vi "test BC + RTs.vi"(8 "error in":errorcluster, 11 "TestCase in":refnum<class "Create Execution Unit.lvclass">) -> (0 "error out":errorcluster, 3 "TestCase out":refnum<class "Create Execution Unit.lvclass">)   [LabVIEW 2023, in "Create Execution Unit.lvclass"]
uses:
  Create Execution Unit.lvclass
  C:/Program Files/National Instruments/LabVIEW 2023/vi.lib/NI/VeriStand Custom Device Testing Tools/VeriStandScriptingTestCase/VeriStandScriptingTestCase.lvclass
  Shared/Map of Messages to Value Indexes.ctl
  Shared/Message Map Key.ctl
  Engine/Implementation/Rx Execution Unit/Message Map Value.ctl
  Shared/Message Definition.ctl
  Shared/Message Type.ctl
  Shared/Terminal Endpoint.ctl
  Shared/Address.ctl
  Shared/Parameter Definition.ctl
  Engine/Implementation/Execution Unit Factory/Execution Unit Factory.lvclass
  Engine/Implementation/Rx Execution Unit/Rx Execution Unit.lvclass
  Engine/Custom Device/Logging Configuration.ctl
  Shared/Data Word Format.ctl
  Shared/Device Parameters.ctl
  Shared/Initialization Method.ctl
  <vilib>/NI/VeriStand Custom Device Testing Tools/VeriStandScriptingTestCase/VeriStandScriptingTestCase.lvclass/VeriStandScriptingTestCase.ctl
  Engine/Implementation/Rx Execution Unit/Rx Execution Unit.lvclass/Rx Execution Unit.ctl
  <vilib>/NI/VeriStand Custom Device Testing Tools/VeriStandScriptingTestCase/Read Target.vi
  Engine/Implementation/Shared Resources/Shared Resources.lvclass
  C:/dev/niveristand-ballard-milStd1553-custom-device/Source/Custom Device Support/Engine/Interfaces/Shared Resources/Shared Resources.lvclass
  NationalInstruments.VeriStand.SystemDefinitionAPI
  Create Execution Unit.lvclass/Create Execution Unit.ctl
  <vilib>/addons/_JKI Toolkits/VI Tester/TestCase.llb/TestCase.lvclass
  Scripting/Ballard MIL-STD-1553 Scripting.lvlib
  Engine/Custom Device/Custom Device.lvlib
  C:/Program Files/National Instruments/LabVIEW 2023/vi.lib/addons/_JKI Toolkits/VI Tester/TestCase.llb/TestCase.lvclass
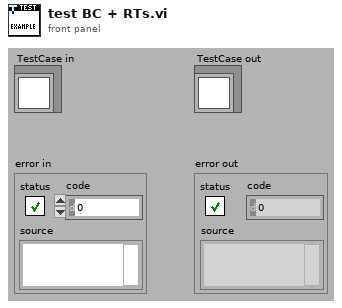
[diagram p1: front panel]
types:
  T1 = typedef "Map of Messages to Value Indexes.ctl" = map{T2, T3}
  T2 = typedef "Message Map Key.ctl" = cluster{"HW channel":u16, "terminal address":u16, "subaddress":u16, "mode code":u16}
  T3 = typedef "Ballard MIL-STD-1553 Engine Support.lvlib/Implementation.lvlib/Rx Execution Unit.lvclass/Message Map Value.ctl" = cluster{"value indexes":i32[], "message":T4, "Tx status count":i32, "Rx status count":i32}
  T4 = typedef "Message Definition.ctl" = cluster{"name":string, "message type":T5, "endpoint Tx":T6, "endpoint Rx":T6, "create timestamp channel":bool, "mode code":u16, "number of words":u16, "parameters":cluster{"name":string, "default value":dbl, "unit":string, "parameter definition":T8}[]}
  T5 = typedef "Message Type.ctl" = string
  T6 = typedef "Terminal Endpoint.ctl" = cluster{"terminal address":T7, "subaddress":T7}
  T7 = typedef "Address.ctl" = u16
  T8 = typedef "Parameter Definition.ctl" = cluster{"start index":i32, "size (bits)":i32, "encoding":enum16{"BNR", "BCD", "Discrete"}, "signed":bool, "multiplier":dbl, "offset":dbl}
  T9 = typedef "Device Parameters.ctl" = cluster{"initialization method":T10, "card number":i32, "PXI slot number":i32, "core number":i32}
  T10 = typedef "Initialization Method.ctl" = enum16{"PXI Slot Number", "Card Number"}
  T11 = typedef "Ballard MIL-STD-1553 Engine Support.lvlib/Custom Device.lvlib/Logging Configuration.ctl" = cluster{"configured":bool, "directory":string, "file name":string, "timestamp file name":bool, "data word format":T12}
  T12 = typedef "Data Word Format.ctl" = string
  T13 = cluster{"Hardware File":path, "Parameters File":path}
  T14 = typedef "Custom Device API.lvlib/Custom Device Item Ref.ctl" = u64
  T15 = typedef "Ballard MIL-STD-1553 Engine Support.lvlib/Interfaces.lvlib/Execution Unit Information.ctl" = cluster{"Execution Unit":refnum<class "Execution Unit.lvclass">, "Incoming Channels":T14[], "Outgoing Channels":T14[], "ReadWrite Channels":T14[]}
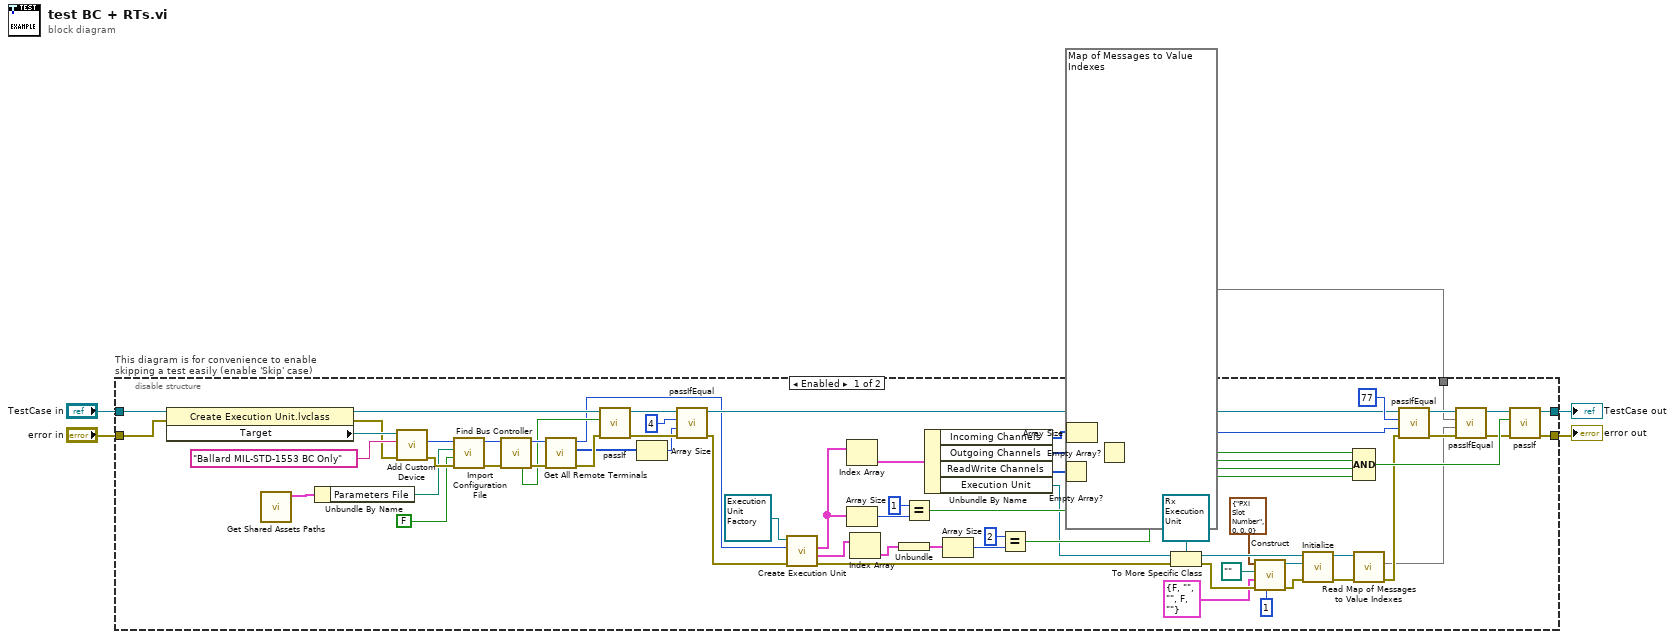
[diagram p0: block diagram]
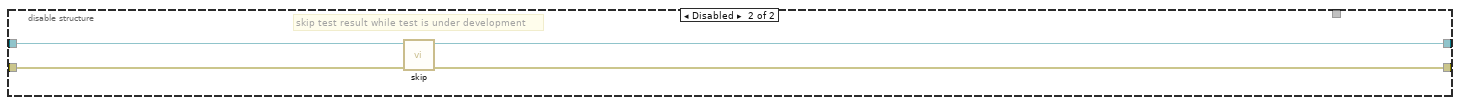
[diagram p2: hidden frame]
diagram:
  n1 = disable-structure "This diagram is for convenience to enable skipping a test easily (enable 'Skip' case)" shown="Enabled" {
    disable-tunnel: "TestCase in" -> [w67 w76]
    disable-tunnel: [w42 w74] -> w2
    disable-tunnel: [w41 w75] -> w4
    disable-tunnel: "error in" -> [w71 w73]
    disable-tunnel: T1 {{"HW channel"=0, "terminal address"=0, "subaddress"=2, "mode code"=0}={"value indexes"=[0], "message"={"name"="BC to RT 0.2", "message type"="BC to RT", "endpoint Tx"={"terminal address"=99, "subaddress"=0}, "endpoint Rx"={"terminal address"=0, "subaddress"=2}, "create timestamp channel"=TRUE, "mode code"=0, "number of words"=3, "parameters"=[{"name"="Word 00", "default value"=0.0, "unit"="", "parameter definition"={"start index"=0, "size (bits)"=16, "encoding"=enum."BNR", "signed"=FALSE, "multiplier"=1.0, "offset"=0.0}}, {"name"="Word 01", "default value"=0.0, "unit"="", "parameter definition"={"start index"=16, "size (bits)"=16, "encoding"=enum."BNR", "signed"=FALSE, "multiplier"=1.0, "offset"=0.0}}, {"name"="Word 02", "default value"=0.0, "unit"="", "parameter definition"={"start index"=32, "size (bits)"=16, "encoding"=enum."BNR", "signed"=FALSE, "multiplier"=1.0, "offset"=0.0}}]}, "Tx status count"=0, "Rx status count"=1}, {"HW channel"=0, "terminal address"=0, "subaddress"=3, "mode code"=0}={"value indexes"=[5], "message"={"name"="BC to RT 0.3", "message type"="BC to RT", "endpoint Tx"={"terminal address"=99, "subaddress"=0}, "endpoint Rx"={"terminal address"=0, "subaddress"=3}, "create timestamp channel"=FALSE, "mode code"=0, "number of words"=4, "parameters"=[{"name"="Word 00", "default value"=0.0, "unit"="", "parameter definition"={"start index"=0, "size (bits)"=16, "encoding"=enum."BNR", "signed"=FALSE, "multiplier"=1.0, "offset"=0.0}}, {"name"="Word 01", "default value"=0.0, "unit"="", "parameter definition"={"start index"=16, "size (bits)"=16, "encoding"=enum."BNR", "signed"=FALSE, "multiplier"=1.0, "offset"=0.0}}, {"name"="Word 02", "default value"=0.0, "unit"="", "parameter definition"={"start index"=32, "size (bits)"=16, "encoding"=enum."BNR", "signed"=FALSE, "multiplier"=1.0, "offset"=0.0}}, {"name"="Word 03", "default value"=0.0, "unit"="", "parameter definition"={"start index"=48, "size (bits)"=16, "encoding"=enum."BNR", "signed"=FALSE, "multiplier"=1.0, "offset"=0.0}}]}, "Tx status count"=0, "Rx status count"=1}, {"HW channel"=0, "terminal address"=0, "subaddress"=5, "mode code"=0}={"value indexes"=[32], "message"={"name"="RT 0.5 to BC", "message type"="RT to BC", "endpoint Tx"={"terminal address"=0, "subaddress"=5}, "endpoint Rx"={"terminal address"=99, "subaddress"=0}, "create timestamp channel"=FALSE, "mode code"=0, "number of words"=6, "parameters"=[{"name"="Word 00", "default value"=0.0, "unit"="", "parameter definition"={"start index"=0, "size (bits)"=16, "encoding"=enum."BNR", "signed"=FALSE, "multiplier"=1.0, "offset"=0.0}}, {"name"="Word 01", "default value"=0.0, "unit"="", "parameter definition"={"start index"=16, "size (bits)"=16, "encoding"=enum."BNR", "signed"=FALSE, "multiplier"=1.0, "offset"=0.0}}, {"name"="Word 02", "default value"=0.0, "unit"="", "parameter definition"={"start index"=32, "size (bits)"=16, "encoding"=enum."BNR", "signed"=FALSE, "multiplier"=1.0, "offset"=0.0}}, {"name"="Word 03", "default value"=0.0, "unit"="", "parameter definition"={"start index"=48, "size (bits)"=16, "encoding"=enum."BNR", "signed"=FALSE, "multiplier"=1.0, "offset"=0.0}}, {"name"="Word 04", "default value"=0.0, "unit"="", "parameter definition"={"start index"=64, "size (bits)"=16, "encoding"=enum."BNR", "signed"=FALSE, "multiplier"=1.0, "offset"=0.0}}, {"name"="Word 05", "default value"=0.0, "unit"="", "parameter definition"={"start index"=80, "size (bits)"=16, "encoding"=enum."BNR", "signed"=FALSE, "multiplier"=1.0, "offset"=0.0}}]}, "Tx status count"=1, "Rx status count"=0}, {"HW channel"=0, "terminal address"=0, "subaddress"=6, "mode code"=0}={"value indexes"=[39], "message"={"name"="RT 0.6 to BC", "message type"="RT to BC", "endpoint Tx"={"terminal address"=0, "subaddress"=6}, "endpoint Rx"={"terminal address"=99, "subaddress"=0}, "create timestamp channel"=TRUE, "mode code"=0, "number of words"=2, "parameters"=[{"name"="Word 00", "default value"=0.0, "unit"="", "parameter definition"={"start index"=0, "size (bits)"=16, "encoding"=enum."BNR", "signed"=FALSE, "multiplier"=1.0, "offset"=0.0}}, {"name"="Word 01", "default value"=0.0, "unit"="", "parameter definition"={"start index"=16, "size (bits)"=16, "encoding"=enum."BNR", "signed"=FALSE, "multiplier"=1.0, "offset"=0.0}}]}, "Tx status count"=1, "Rx status count"=0}, {"HW channel"=0, "terminal address"=0, "subaddress"=31, "mode code"=16}={"value indexes"=[16], "message"={"name"="MC 16", "message type"="MC", "endpoint Tx"={"terminal address"=0, "subaddress"=31}, "endpoint Rx"={"terminal address"=99, "subaddress"=0}, "create timestamp channel"=FALSE, "mode code"=16, "number of words"=1, "parameters"=[{"name"="Word 00", "default value"=0.0, "unit"="", "parameter definition"={"start index"=0, "size (bits)"=16, "encoding"=enum."BNR", "signed"=FALSE, "multiplier"=1.0, "offset"=0.0}}]}, "Tx status count"=1, "Rx status count"=0}, {"HW channel"=0, "terminal address"=0, "subaddress"=31, "mode code"=17}={"value indexes"=[18], "message"={"name"="MC 17", "message type"="MC", "endpoint Tx"={"terminal address"=99, "subaddress"=0}, "endpoint Rx"={"terminal address"=0, "subaddress"=31}, "create timestamp channel"=FALSE, "mode code"=17, "number of words"=1, "parameters"=[{"name"="Word 00", "default value"=0.0, "unit"="", "parameter definition"={"start index"=0, "size (bits)"=16, "encoding"=enum."BNR", "signed"=FALSE, "multiplier"=1.0, "offset"=0.0}}]}, "Tx status count"=0, "Rx status count"=1}, {"HW channel"=0, "terminal address"=15, "subaddress"=20, "mode code"=0}={"value indexes"=[20, 26], "message"={"name"="RT 0.20 to RT 15.20", "message type"="RT to RT", "endpoint Tx"={"terminal address"=0, "subaddress"=20}, "endpoint Rx"={"terminal address"=15, "subaddress"=20}, "create timestamp channel"=FALSE, "mode code"=0, "number of words"=4, "parameters"=[{"name"="Word 00", "default value"=0.0, "unit"="", "parameter definition"={"start index"=0, "size (bits)"=16, "encoding"=enum."BNR", "signed"=FALSE, "multiplier"=1.0, "offset"=0.0}}, {"name"="Word 01", "default value"=0.0, "unit"="", "parameter definition"={"start index"=16, "size (bits)"=16, "encoding"=enum."BNR", "signed"=FALSE, "multiplier"=1.0, "offset"=0.0}}, {"name"="Word 02", "default value"=0.0, "unit"="", "parameter definition"={"start index"=32, "size (bits)"=16, "encoding"=enum."BNR", "signed"=FALSE, "multiplier"=1.0, "offset"=0.0}}, {"name"="Word 03", "default value"=0.0, "unit"="", "parameter definition"={"start index"=48, "size (bits)"=16, "encoding"=enum."BNR", "signed"=FALSE, "multiplier"=1.0, "offset"=0.0}}]}, "Tx status count"=1, "Rx status count"=1}, {"HW channel"=0, "terminal address"=31, "subaddress"=21, "mode code"=0}={"value indexes"=[43, 54], "message"={"name"="RT 15.21 to RT 31.21", "message type"="RT to RT", "endpoint Tx"={"terminal address"=15, "subaddress"=21}, "endpoint Rx"={"terminal address"=31, "subaddress"=21}, "create timestamp channel"=TRUE, "mode code"=0, "number of words"=11, "parameters"=[{"name"="Parameter 0", "default value"=0.0, "unit"="", "parameter definition"={"start index"=0, "size (bits)"=16, "encoding"=enum."BNR", "signed"=FALSE, "multiplier"=2.0, "offset"=0.0}}, {"name"="Parameter 1", "default value"=0.0, "unit"="", "parameter definition"={"start index"=16, "size (bits)"=16, "encoding"=enum."BNR", "signed"=FALSE, "multiplier"=1.0, "offset"=50.0}}, {"name"="Parameter 2", "default value"=0.0, "unit"="", "parameter definition"={"start index"=32, "size (bits)"=16, "encoding"=enum."BNR", "signed"=TRUE, "multiplier"=1.0, "offset"=0.0}}, {"name"="Parameter 3", "default value"=0.0, "unit"="", "parameter definition"={"start index"=48, "size (bits)"=16, "encoding"=enum."BNR", "signed"=FALSE, "multiplier"=1.0, "offset"=0.0}}, {"name"="Parameter 4", "default value"=0.0, "unit"="", "parameter definition"={"start index"=64, "size (bits)"=16, "encoding"=enum."BNR", "signed"=FALSE, "multiplier"=1.0, "offset"=0.0}}, {"name"="Parameter 5", "default value"=0.0, "unit"="", "parameter definition"={"start index"=80, "size (bits)"=16, "encoding"=enum."BNR", "signed"=FALSE, "multiplier"=1.0, "offset"=0.0}}, {"name"="Parameter 6", "default value"=0.0, "unit"="", "parameter definition"={"start index"=96, "size (bits)"=32, "encoding"=enum."BNR", "signed"=FALSE, "multiplier"=1.0, "offset"=0.0}}, {"name"="Parameter 8", "default value"=0.0, "unit"="", "parameter definition"={"start index"=128, "size (bits)"=8, "encoding"=enum."BNR", "signed"=TRUE, "multiplier"=1.0, "offset"=0.0}}, {"name"="Parameter 9", "default value"=0.0, "unit"="", "parameter definition"={"start index"=136, "size (bits)"=40, "encoding"=enum."BNR", "signed"=FALSE, "multiplier"=1.0, "offset"=0.0}}]}, "Tx status count"=1, "Rx status count"=0}, {"HW channel"=0, "terminal address"=31, "subaddress"=28, "mode code"=0}={"value indexes"=[10], "message"={"name"="BC to RT 31.28", "message type"="BC to RT", "endpoint Tx"={"terminal address"=99, "subaddress"=0}, "endpoint Rx"={"terminal address"=31, "subaddress"=28}, "create timestamp channel"=FALSE, "mode code"=0, "number of words"=6, "parameters"=[{"name"="Word 00", "default value"=0.0, "unit"="", "parameter definition"={"start index"=0, "size (bits)"=16, "encoding"=enum."BNR", "signed"=FALSE, "multiplier"=1.0, "offset"=0.0}}, {"name"="Word 01", "default value"=0.0, "unit"="", "parameter definition"={"start index"=16, "size (bits)"=16, "encoding"=enum."BNR", "signed"=FALSE, "multiplier"=1.0, "offset"=0.0}}, {"name"="Word 02", "default value"=0.0, "unit"="", "parameter definition"={"start index"=32, "size (bits)"=16, "encoding"=enum."BNR", "signed"=FALSE, "multiplier"=1.0, "offset"=0.0}}, {"name"="Word 03", "default value"=0.0, "unit"="", "parameter definition"={"start index"=48, "size (bits)"=16, "encoding"=enum."BNR", "signed"=FALSE, "multiplier"=1.0, "offset"=0.0}}, {"name"="Word 04", "default value"=0.0, "unit"="", "parameter definition"={"start index"=64, "size (bits)"=16, "encoding"=enum."BNR", "signed"=FALSE, "multiplier"=1.0, "offset"=0.0}}, {"name"="Word 05", "default value"=0.0, "unit"="", "parameter definition"={"start index"=80, "size (bits)"=16, "encoding"=enum."BNR", "signed"=FALSE, "multiplier"=1.0, "offset"=0.0}}]}, "Tx status count"=0, "Rx status count"=0}, {"HW channel"=0, "terminal address"=31, "subaddress"=31, "mode code"=1}={"value indexes"=[], "message"={"name"="MC 01", "message type"="MC", "endpoint Tx"={"terminal address"=99, "subaddress"=0}, "endpoint Rx"={"terminal address"=31, "subaddress"=31}, "create timestamp channel"=FALSE, "mode code"=1, "number of words"=0, "parameters"=[]}, "Tx status count"=0, "Rx status count"=0}} ("map of messages to value indexes") -> [w7 _]
    frame Enabled {
      n2 = property class="Create Execution Unit.lvclass"(reference=w67, error in=w71) -> (reference out=w72:refnum<class "Create Execution Unit.lvclass">, error out=w68:errorcluster, "Target"=w69:refnum<k24>)
      n3 = call "Get Shared Assets Paths.vi"() -> ("BC and RTs"=w13:T13)  [unwired: 9 in, 2 out]
      n4 = Unbundle By Name(w13) -> ("Parameters File"=w12:path)
      n5 = call "Add Custom Device.vi"("error in"=w68, "name"="Ballard MIL-STD-1553 BC Only", "target in"=w69) -> ("error out"=w16:errorcluster, "Ballard MIL-STD 1553 custom device"=w17:T14)  [unwired: 6 in, 1 out]
      n6 = call "Import Configuration File.vi"("error in"=w16, "create Tx/Rx folders for subaddresses?"=FALSE, "parameters configuration file path"=w12, "Ballard MIL-STD 1553 custom device in"=w17) -> ("error out"=w14:errorcluster, "Ballard MIL-STD 1553 custom device out"=w15:T14)  [unwired: 6 in]
      n7 = call "Find Bus Controller.vi"("error in"=w14, "port in"=w15) -> ("error out"=w57:errorcluster, "port out"=w58:T14, "found?"=w56:bool)  [unwired: 6 in, 1 out]
      n8 = call "Get All Remote Terminals.vi"("error in"=w57, "port in"=w58) -> ("error out"=w55:errorcluster, "remote terminals"=w54:T14[], "port out"=w23:T14)  [unwired: 7 in]
      n9 = call-dynamic "passIf.vi"("error in (no error)"=w55, "pass"=w56, "TestCase in"=w72) -> ("error out"=w60:errorcluster, "TestCase out"=w61:refnum<class "Create Execution Unit.lvclass">)  [unwired: 7 in]
      n10 = Array Size(array=w54) -> (size(s)=w53:i32)
      n11 = call-dynamic "passIfEqual.vi"("error in (no error)"=w60, "y"=w53, "x"=4 ("size(s)"), "TestCase in"=w61) -> ("error out"=w59:errorcluster, "TestCase out"=w45:refnum<class "Create Execution Unit.lvclass">)  [unwired: 6 in]
      n12 = call-dynamic "Create Execution Unit.vi"("error in"=w59, "Item Ref"=w23, "Execution Unit Factory Implementation in"=refnum<class "Execution Unit Factory.lvclass"> refnum) -> ("error out"=w35:errorcluster, "Asynchronous Execution Units"=w11:cluster{"Grouped Execution Units":T15[]}[], "Inline Execution Units"=w51:T15[])  [unwired: 5 in, 1 out]
      n13 = Index Array(array=w51) -> (element=w50:T15)  [unwired: 1 in]
      n14 = Array Size(array=w51) -> (size(s)=w65:i32)
      n15 = Index Array(array=w11) -> (element=w10:cluster{"Grouped Execution Units":T15[]})  [unwired: 1 in]
      n16 = Unbundle(w10) -> ("Grouped Execution Units"=w9:T15[])
      n17 = Equal?(x=1, y=w65) -> (x = y?=w44:bool)
      n18 = Unbundle By Name(w50) -> ("Incoming Channels"=w49:T14[], "Outgoing Channels"=w21:T14[], "ReadWrite Channels"=w19:T14[], "Execution Unit"=w36:refnum<class "Execution Unit.lvclass">)
      n19 = Array Size(array=w9) -> (size(s)=w64:i32)
      n20 = Equal?(x=2, y=w64) -> (x = y?=w43:bool)
      n21 = Empty Array?(array=w19) -> (empty?=w18:bool)
      n22 = Array Size(array=w49) -> (size(s)=w47:i32)
      n23 = Empty Array?(array=w21) -> (empty?=w20:bool)
      n24 = To More Specific Class(target class=refnum<class "Rx Execution Unit.lvclass"> refnum ("Rx execution unit in"), reference=w36, error in=w35) -> (specific class reference=w37:refnum<class "Rx Execution Unit.lvclass">, error out=w32:errorcluster)
      n25 = call "Construct.vi"("number of ports"=1, "error in"=w32, "logging configuration"=T11 {"configured"=FALSE, "directory"="", "file name"="", "timestamp file name"=FALSE, "data word format"=""}, "hardware config file"=path "", "device parameters"=T9 {"initialization method"=enum."PXI Slot Number", "card number"=0, "PXI slot number"=0, "core number"=0}) -> ("error out"=w31:errorcluster, "Ballard 1553 shared resources"=w34:refnum<class "Shared Resources.lvclass">)  [unwired: 5 in]
      n26 = call-dynamic "Initialize.vi"("error in"=w31, "shared resources"=w34, "Rx Execution Unit Implementation in"=w37) -> ("error out"=w22:errorcluster, "Rx Execution Unit Implementation out"=w38:refnum<class "Rx Execution Unit.lvclass">)  [unwired: 7 in]
      n27 = Compound Arithmetic op=AND(w20, w18, w44, w43) -> (w48:bool)
      n28 = call "Read Map of Messages to Value Indexes.vi"("error in"=w22, "Rx execution unit in"=w38) -> ("error out"=w39:errorcluster, "map of messages to value indexes"=w8:T1)  [unwired: 7 in, 1 out]
      n29 = call-dynamic "passIfEqual.vi"("error in (no error)"=w39, "y"=w47, "x"=77 ("size(s)"), "TestCase in"=w45) -> ("error out"=w27:errorcluster, "TestCase out"=w26:refnum<class "Create Execution Unit.lvclass">)  [unwired: 6 in]
      n30 = call-dynamic "passIfEqual.vi"("error in (no error)"=w27, "y"=w8, "x"=w7, "TestCase in"=w26) -> ("error out"=w24:errorcluster, "TestCase out"=w25:refnum<class "Create Execution Unit.lvclass">)  [unwired: 6 in]
      n31 = call-dynamic "passIf.vi"("error in (no error)"=w24, "pass"=w48, "TestCase in"=w25) -> ("error out"=w41:errorcluster, "TestCase out"=w42:refnum<class "Create Execution Unit.lvclass">)  [unwired: 7 in]
    }
    frame Disabled {
      # "skip test result while test is under development"
      n32 = call <vilib>:"skip.vi"("error in (no error)"=w73, "TestCase in"=w76) -> ("error out"=w75:errorcluster, "TestCase out"=w74:refnum<class "Create Execution Unit.lvclass">)  [unwired: 8 in]
    }
  }
  "error out" <- w4
  "TestCase out" <- w2
